vi "RT-Main (inventory only).vi"() -> ()   [LabVIEW 2016]
uses:
  <vilib>/NI_Real-Time Target Support.lvlib
  Inventory FGV Command.ctl
  Update Screen.ctl
panel:
  in  "Stop Button 2":bool
  in  "Stop Button":bool
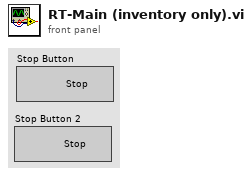
[diagram p1: front panel]
types:
  T1 = typedef "Update Screen.ctl" = cluster{"Time":string, "Item":string, "Name":string, "Action":string, "Lunch Names":string[]}
  T2 = typedef "Inventory FGV Command.ctl" = enum16{"Load Items", "Check Status", "Return Items", "Check Out Items", "Add New Item", "Get All Items", "Remove Item", "Search"}
  T3 = typedef "Array Device Info.ctl" = T4[]
  T4 = typedef "Device Info.ctl" = cluster{"Model Number":string, "Identifier":string, "Available?":bool, "Owner":string, "Owner Email":string, "Last Activity Date":string, "Loan Purpose":string, "Department":string, "Notes":string, "Serial Number":string}
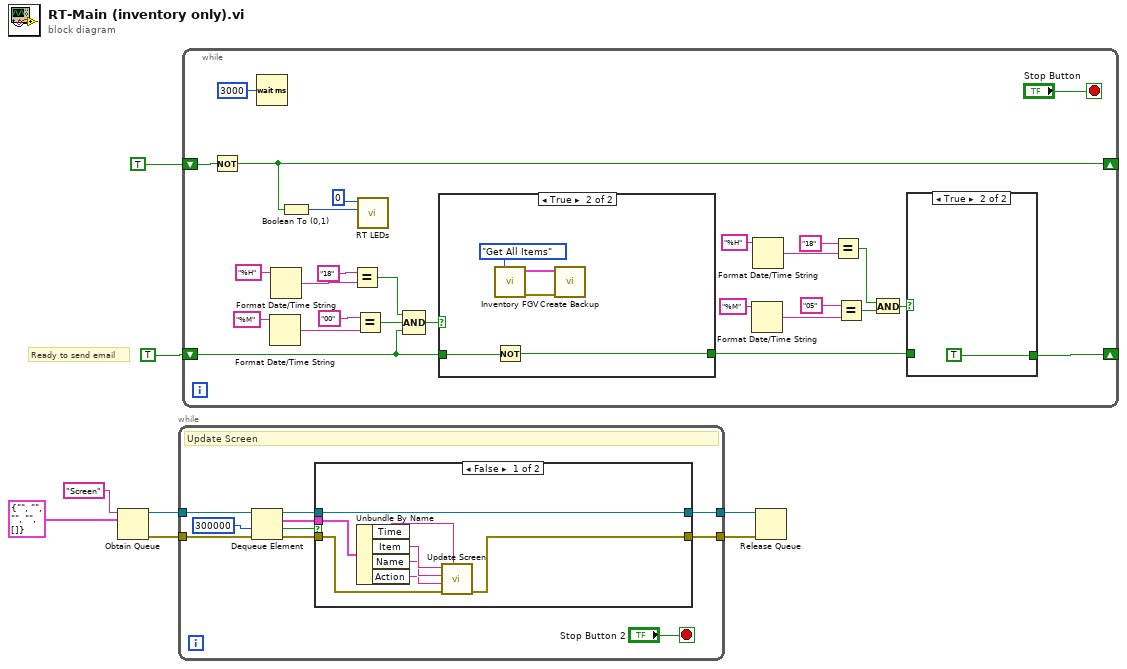
[diagram p0: block diagram]
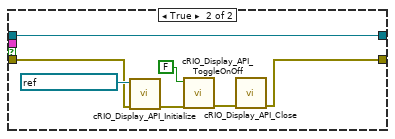
[diagram p2: hidden frame]
diagram:
  # "Ready to send email"
  n1 = Obtain Queue(name (unnamed)="Screen", element data type=T1 {"Time"="", "Item"="", "Name"="", "Action"="", "Lunch Names"=[]}) -> (queue out=w5:refnum<queue>, error out=w4:errorcluster)  [unwired: 3 in, 1 out]
  n2 = while {
    tunnel: w5 -> [w17]
    tunnel: w4 -> [w16]
    tunnel: [w10] -> w2
    tunnel: [w9] -> w1
    stop <- "Stop Button 2" stop-if-true
    # "Update Screen"
    n3 = Dequeue Element(queue=w17, timeout in ms (-1)=300000, error in (no error)=w16) -> (queue out=w11:refnum<queue>, element=w12:T1, timed out?=w14:bool, error out=w13:errorcluster)
    n4 = case shown="False" w14 {
      tunnel: w13 -> [w26 w29]
      tunnel: w12 -> [w23 _]
      tunnel: w11 -> [w24 w33]
      tunnel: [w25 w28] -> w10
      tunnel: [w24 w33] -> w9
      frame False {
        n5 = Unbundle By Name(w23) -> ("Time"=w22:string, "Item"=w21:string, "Name"=w20:string, "Action"=w19:string)
        n6 = call "Update Screen.vi"(7:w22, "error in (no error)"=w26, 9:w19, 10:w20, "Update Screen"=w21) -> ("error out"=w25:errorcluster)  [unwired: 6 in]
      }
      frame True {
        n7 = call <vilib>:"cRIO_Display_API_Initialize.vi"("error in"=w29, "cRIODisplay Port"=refnum<visa-resource-name> "ASRL1::INSTR") -> ("error out"=w32:errorcluster)  [unwired: 9 in]
        n8 = call <vilib>:"cRIO_Display_API_ToggleOnOff.vi"("error in"=w32, "On/Off"=FALSE) -> ("error out"=w31:errorcluster)  [unwired: 9 in]
        n9 = call <vilib>:"cRIO_Display_API_Close.vi"("error in"=w31) -> ("error out"=w28:errorcluster)  [unwired: 10 in]
      }
    }
  }
  n10 = while {
    shift-right: [w58] -> _
    shift-left: TRUE -> [w59]
    shift-right: [w34] -> _
    shift-left: TRUE -> [w45]
    stop <- "Stop Button" stop-if-true
    n11 = Not(x=w59) -> (.not. x?=w58:bool)
    n12 = Wait (ms)(milliseconds to wait=u32 3000) -> ()  [unwired: 1 out]
    n13 = Format Date/Time String(time format string (%c)="%M") -> (date/time string=w50:string)  [unwired: 2 in]
    n14 = Format Date/Time String(time format string (%c)="%H") -> (date/time string=w52:string)  [unwired: 2 in]
    n15 = Boolean To (0,1)(Boolean=w58) -> (0, 1=w57:i16)
    n16 = Equal?(x="18", y=w52) -> (x = y?=w48:bool)
    n17 = Equal?(x="00", y=w50) -> (x = y?=w47:bool)
    n18 = call <vilib>:"RT LEDs.vi"("State"=w57, "LED Num"=0) -> ()  [unwired: 4 in, 2 out]
    n19 = Compound Arithmetic op=AND(w48, w47, w45) -> (w46:bool)
    n20 = case shown="True" w46 {
      tunnel: w45 -> [w61 w66]
      tunnel: [w61 w65] -> w35
      frame False {
      }
      frame True {
        n21 = call "Inventory FGV.vi"("Command"=Inventory_FGV_Command."Get All Items") -> ("error out"=w62:errorcluster, "array of devices"=w63:T3)  [unwired: 7 in, 1 out]
        n22 = Not(x=w66) -> (.not. x?=w65:bool)
        n23 = call "Create Backup.vi"("error in"=w62, "array of devices"=w63) -> ()  [unwired: 9 in, 1 out]
      }
    }
    n24 = Format Date/Time String(time format string (%c)="%M") -> (date/time string=w43:string)  [unwired: 2 in]
    n25 = Format Date/Time String(time format string (%c)="%H") -> (date/time string=w41:string)  [unwired: 2 in]
    n26 = Equal?(x="18", y=w41) -> (x = y?=w38:bool)
    n27 = Equal?(x="05", y=w43) -> (x = y?=w37:bool)
    n28 = And(x=w38, y=w37) -> (x .and. y?=w36:bool)
    n29 = case shown="True" w36 {
      tunnel: w35 -> [w67 _]
      tunnel: [w67 TRUE] -> w34
      frame False {
      }
      frame True {
      }
    }
  }
  n30 = Release Queue(queue=w1, error in (no error)=w2) -> ()  [unwired: 1 in, 3 out]
